vi "Build Drag Data.vi"(2 "Source":string, 3 "Mode":string) -> (0 "Drag Data":T1(array[cluster]))   [LabVIEW 2015, in "Editor.lvclass"]
uses:
  Editor.lvclass
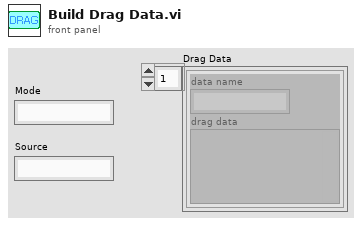
[diagram p1: front panel]
types:
  T1 = cluster{"data name":string, "drag data":variant}[]
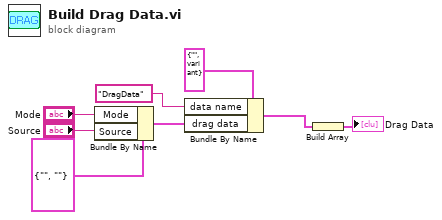
[diagram p0: block diagram]
diagram:
  n1 = Bundle By Name(cluster=cluster{"Mode":string, "Source":string} {"Mode"="", "Source"=""}, "Mode"="Mode", "Source"="Source") -> (w1:cluster{"Mode":string, "Source":string})
  n2 = Bundle By Name(cluster=cluster{"data name":string, "drag data":variant} {"data name"="", "drag data"=variant}, "data name"="DragData", "drag data"=w1) -> (w6:cluster{"data name":string, "drag data":variant})
  n3 = Build Array(w6) -> (→"Drag Data":T1)
